vi "初始化.vi"   [LabVIEW 2022 SP3]
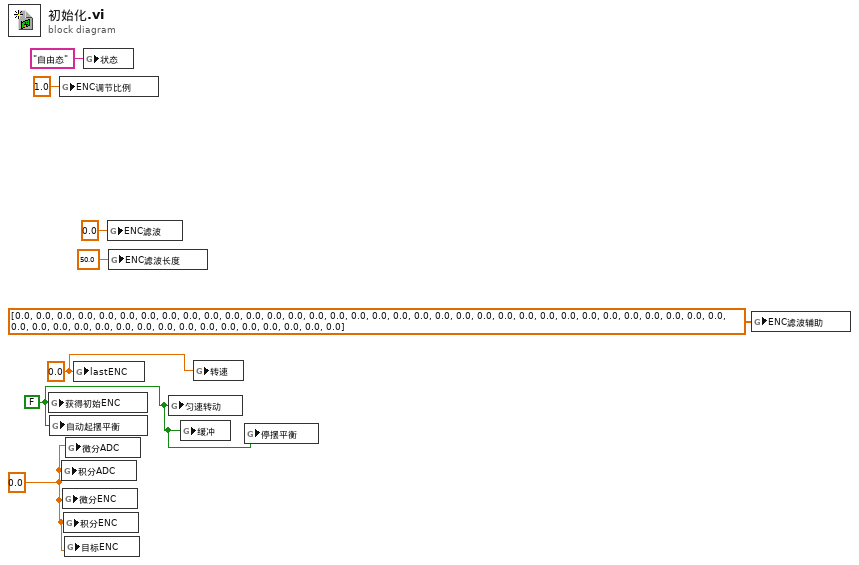
[diagram p0: block diagram]
diagram:
  w3 = 0.0 ("积分ADC")
  w1 = FALSE ("获得初始ENC")
  w2 = 0.0 ("lastENC")
  n1 = global write "全局变量.vi" "获得初始ENC"(w1) -> ()
  n2 = global write "全局变量.vi" "自动起摆平衡"(w1) -> ()
  n3 = global write "全局变量.vi" "ENC调节比例"(1.0 ("ENC调节比例")) -> ()
  n4 = global write "全局变量.vi" "积分ADC"(w3) -> ()
  n5 = global write "全局变量.vi" "微分ENC"(w3) -> ()
  n6 = global write "全局变量.vi" "积分ENC"(w3) -> ()
  n7 = global write "全局变量.vi" "目标ENC"(w3) -> ()
  n8 = global write "全局变量.vi" "微分ADC"(w3) -> ()
  n9 = global write "全局变量.vi" "lastENC"(w2) -> ()
  n10 = global write "全局变量.vi" "状态"("自由态" ("状态")) -> ()
  n11 = global write "全局变量.vi" "ENC滤波"(0.0 ("ENC滤波")) -> ()
  n12 = global write "全局变量.vi" "ENC滤波长度"(50.0 ("ENC滤波长度")) -> ()
  n13 = global write "全局变量.vi" "匀速转动"(w1) -> ()
  n14 = global write "全局变量.vi" "缓冲"(w1) -> ()
  n15 = global write "全局变量.vi" "转速"(w2) -> ()
  n16 = global write "全局变量.vi" "停摆平衡"(w1) -> ()
  n17 = global write "全局变量.vi" "ENC滤波辅助"(dbl[] [0.0, 0.0, 0.0, 0.0, 0.0, 0.0, 0.0, 0.0, 0.0, 0.0, 0.0, 0.0, 0.0, 0.0, 0.0, 0.0, 0.0, 0.0, 0.0, 0.0, 0.0, 0.0, 0.0, 0.0, 0.0, 0.0, 0.0, 0.0, 0.0, 0.0, 0.0, 0.0, 0.0, 0.0, 0.0, 0.0, 0.0, 0.0, 0.0, 0.0, 0.0, 0.0, 0.0, 0.0, 0.0, 0.0, 0.0, 0.0, 0.0, 0.0]) -> ()
